vi "json_parse.vi"(8 "error in (no error)":errorcluster, 11 "source":string) -> (0 "error out":errorcluster, 3 "value":variant)   [LabVIEW 2011]
doc: "Parse a JSON message to a set of variant attributes."
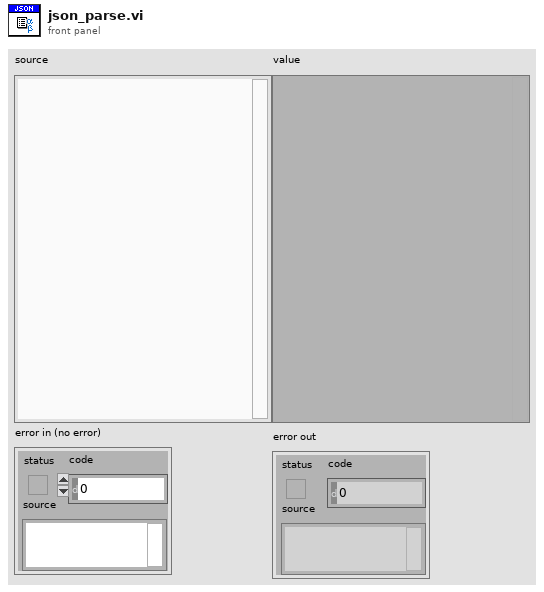
[diagram p1: front panel]
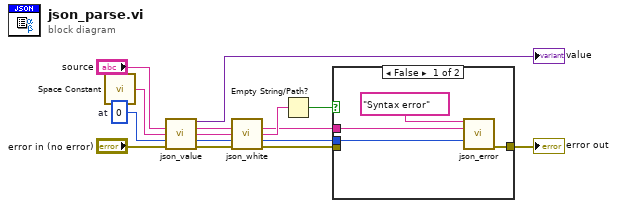
[diagram p0: block diagram]
diagram:
  w13 = 0  # at
  n1 = call <vilib>:"Space Constant.vi"() -> ("String"=w14:string)
  n2 = call "json_value.vi"("text"="source", "ch"=w14, "at"=w13, "error in (no error)"="error in (no error)") -> ("value"=→"value":variant, "text dup"=w11:string, "ch out"=w10:string, "at out"=w9:i32, "error out"=w8:errorcluster)  [unwired: 7 in]
  n3 = call "json_white.vi"("text"=w11, "ch"=w10, "at"=w9, "error in (no error)"=w8) -> ("text dup"=w1:string, "ch out"=w7:string, "at out"=w2:i32, "error out"=w5:errorcluster)  [unwired: 8 in]
  n4 = Empty String/Path?(string/path=w7) -> (empty?=w6:bool)
  n5 = case shown="False" w6 {
    tunnel: [w19 w20] -> w3
    tunnel: w5 -> [_ w20]
    tunnel: w2 -> [w18 _]
    tunnel: w1 -> [w17 _]
    frame False {
      n6 = call "json_error.vi"("m"="Syntax error", "text"=w17, "at"=w18) -> ("error out"=w19:errorcluster)  [unwired: 12 in]
    }
    frame True {
    }
  }
  "error out" <- w3
